vi "Match first tags ASCII and Unicode.vi"(6 "Type":T1, 9 "Hyperlink":string, 11 "Text":string) -> (1 "Array":T3(array[cluster]), 3 "Find tag ?":bool)   [LabVIEW 2019, in "Exaprom PDF.lvlib"]
doc: "Version 1.0\nDeveloped by Jean-Marc Simard\nCopyright © 2010, Exaprom Inc.\nAll rights reserved.\nLicense: BSD"
uses:
  Controls/Text Controls/Text type.ctl
  Controls/Text Controls/Unicode/Character type.ctl
  Exaprom PDF.lvlib
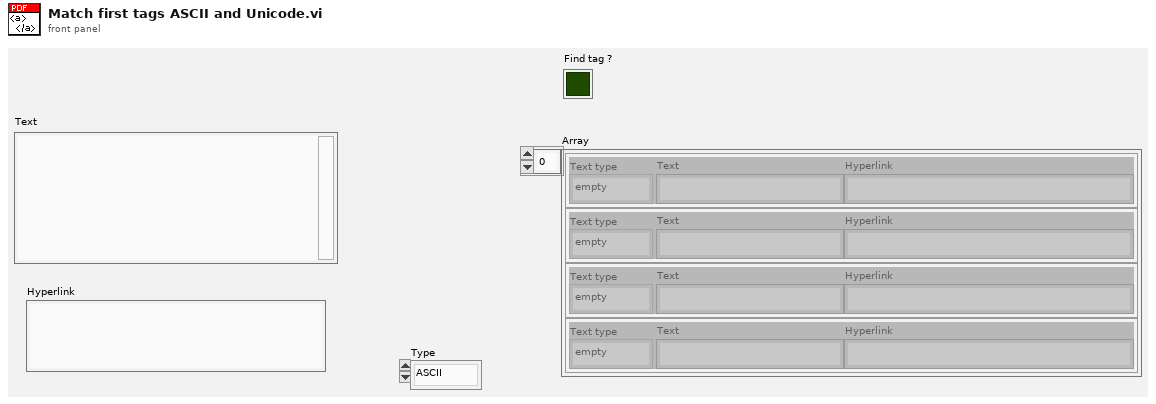
[diagram p1: front panel]
types:
  T1 = typedef "Exaprom PDF.lvlib/Character type.ctl" = enum16{"ASCII", "Unicode"}
  T2 = typedef "Exaprom PDF.lvlib/Text type.ctl" = enum16{"empty", "Text", "Hyperlink"}
  T3 = cluster{"Text type":T2, "Text":string, "Hyperlink":string}[]
  T4 = cluster{"Text type":T2, "Text type":T2, "Text type":T2}
  T5 = cluster{"Text type":T2, "Unicode String OUT":string, "Hyperlink":string}
  T6 = cluster{"Text type":T2, "Unicode String OUT":string, string}
  T7 = cluster{"Text type":T2, "Unicode String OUT":string, "Hyperlink":string}[]
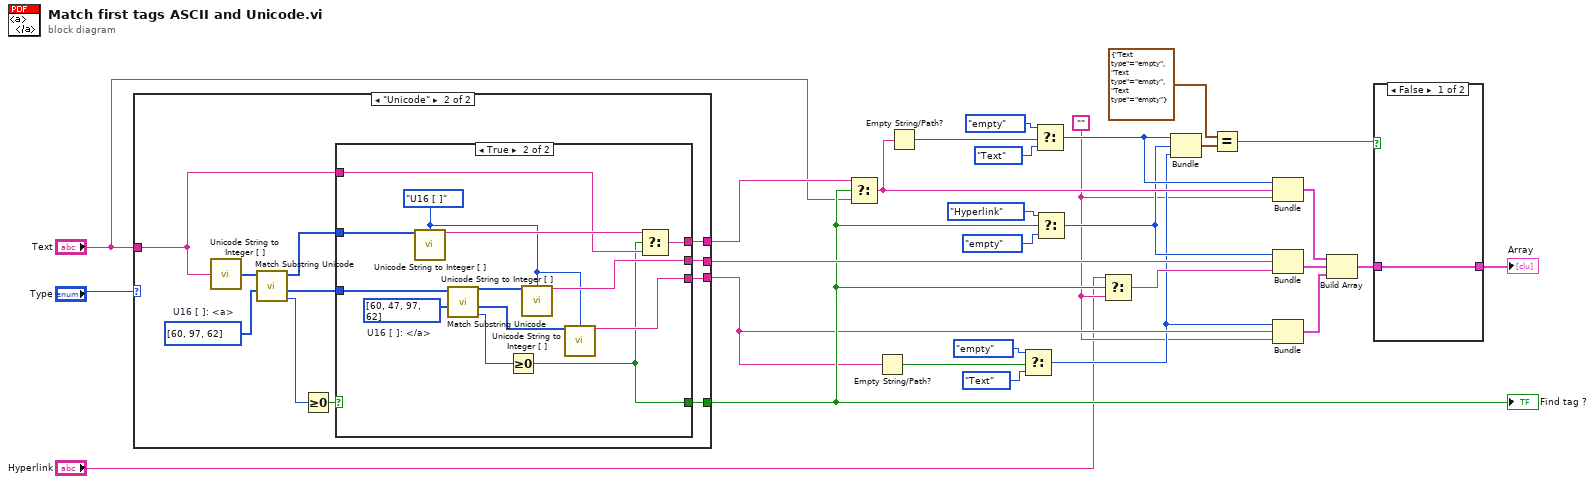
[diagram p0: block diagram]
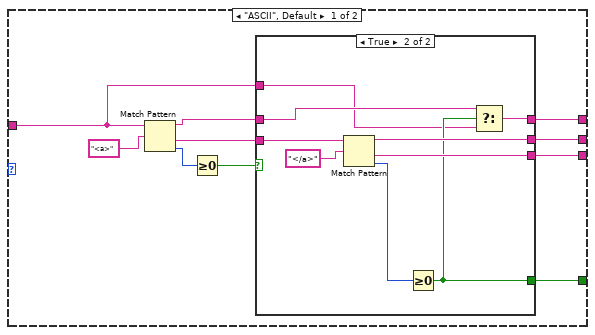
[diagram p2: hidden frame]
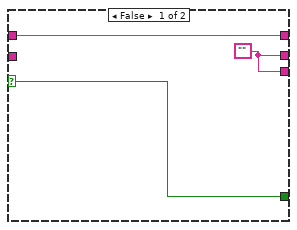
[diagram p3: hidden frame]
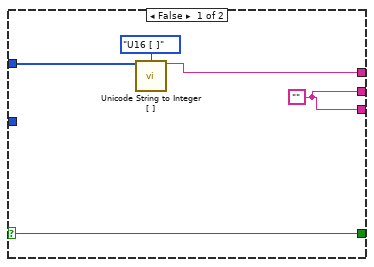
[diagram p4: hidden frame]
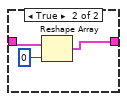
[diagram p5: hidden frame]
diagram:
  w4 = ""
  n1 = case shown="\"Unicode\"" "Type" {
    tunnel: [w34 w54] -> w29
    tunnel: [w33 w53] -> w24
    tunnel: [w32 w52] -> w18
    tunnel: [w31 w56] -> w13
    tunnel: "Text" -> [w30 w55]
    frame "ASCII", Default {
      n2 = Match Pattern(string=w30, regular expression="<a>") -> (before substring=w36:string, after substring=w35:string, offset past match=w39:i32)  [unwired: 2 out]
      n3 = Greater Or Equal To 0?(x=w39) -> (x >= 0?=w38:bool)
      n4 = case shown="True" w38 {
        selector: w38 -> [w40 _]
        tunnel: w36 -> [w42 w44]
        tunnel: [w42 w46] -> w33
        tunnel: w35 -> [_ w51]
        tunnel: [w41 w49] -> w34
        tunnel: [w41 w48] -> w31
        tunnel: [w40 w45] -> w32
        tunnel: w30 -> [_ w43]
        frame False {
          w41 = ""
        }
        frame True {
          n5 = Match Pattern(string=w51, regular expression="</a>") -> (before substring=w49:string, after substring=w48:string, offset past match=w47:i32)  [unwired: 2 out]
          n6 = Greater Or Equal To 0?(x=w47) -> (x >= 0?=w45:bool)
          n7 = Select(t=w44, s=w45, f=w43) -> (s? t:f=w46:string)
        }
      }
    }
    frame "Unicode" {
      w62 = u16[] [60, 97, 62]  # U16 [ ]: <a>
      n8 = call "Unicode String to Integer [ ].vi"("Unicode String"=w55) -> ("Char U16 [ ]"=w57:u16[])  [unwired: 12 in, 2 out]
      n9 = call "Match Substring Unicode.vi"("Substring (U16) [ ]"=w62, "String (U16) [ ]"=w57) -> ("offset past match"=w58:i32, "after substring"=w61:u16[], "before substring"=w60:u16[])  [unwired: 4 in, 1 out]
      n10 = Greater Or Equal To 0?(x=w58) -> (x >= 0?=w59:bool)
      n11 = case shown="True" w59 {
        selector: w59 -> [w66 _]
        tunnel: w60 -> [w64 w80]
        tunnel: w61 -> [_ w78]
        tunnel: w55 -> [_ w76]
        tunnel: [w63 w75] -> w53
        tunnel: [w67 w73] -> w54
        tunnel: [w67 w71] -> w56
        tunnel: [w66 w70] -> w52
        frame False {
          w67 = ""
          n12 = call "Unicode String to Integer [ ].vi"("Char U16 [ ] IN"=w64, "From"=enum16{"String", "U16 [ ]"}."U16 [ ]") -> ("Unicode String OUT"=w63:string)  [unwired: 11 in, 2 out]
        }
        frame True {
          w69 = u16[] [60, 47, 97, 62]  # U16 [ ]: </a>
          w68 = enum16{"String", "U16 [ ]"}."U16 [ ]" ("From")
          n13 = call "Unicode String to Integer [ ].vi"("Char U16 [ ] IN"=w80, "From"=w68) -> ("Unicode String OUT"=w79:string)  [unwired: 11 in, 2 out]
          n14 = call "Match Substring Unicode.vi"("Substring (U16) [ ]"=w69, "String (U16) [ ]"=w78) -> ("offset past match"=w77:i32, "after substring"=w72:u16[], "before substring"=w74:u16[])  [unwired: 4 in, 1 out]
          n15 = Greater Or Equal To 0?(x=w77) -> (x >= 0?=w70:bool)
          n16 = call "Unicode String to Integer [ ].vi"("Char U16 [ ] IN"=w74, "From"=w68) -> ("Unicode String OUT"=w73:string)  [unwired: 11 in, 2 out]
          n17 = call "Unicode String to Integer [ ].vi"("Char U16 [ ] IN"=w72, "From"=w68) -> ("Unicode String OUT"=w71:string)  [unwired: 11 in, 2 out]
          n18 = Select(t=w79, s=w70, f=w76) -> (s? t:f=w75:string)
        }
      }
    }
  }
  "Find tag ?" <- w18
  n19 = Select(t=w24, s=w18, f="Text") -> (s? t:f=w17:string)
  n20 = Empty String/Path?(string/path=w13) -> (empty?=w14:bool)
  n21 = Empty String/Path?(string/path=w17) -> (empty?=w23:bool)
  n22 = Select(t=Text_type."empty" ("Text type"), s=w14, f=Text_type."Text" ("Text type")) -> (s? t:f=w10:T2)
  n23 = Select(t=Text_type."empty" ("Text type"), s=w23, f=Text_type."Text" ("Text type")) -> (s? t:f=w12:T2)
  n24 = Select(t=Text_type."Hyperlink" ("Text type"), s=w18, f=Text_type."empty" ("Text type")) -> (s? t:f=w11:T2)
  n25 = Select(t="Hyperlink", s=w18, f=w4) -> (s? t:f=w28:string)
  n26 = Bundle("Text type"=w12, "Text type"=w11, "Text type"=w10) -> (w9:T4)  [unwired: 1 out]
  n27 = Equal?(x=T4 {"Text type"=enum."empty", "Text type"=enum."empty", "Text type"=enum."empty"}, y=w9) -> (x = y?=w7:bool)
  n28 = Bundle("Text type"=w12, "Text"=w17, w4) -> (w27:cluster{"Text type":T2, "Text":string, string})  [unwired: 1 out]
  n29 = Bundle("Text type"=w11, "Unicode String OUT"=w29, "Hyperlink"=w28) -> (w26:T5)  [unwired: 1 out]
  n30 = Bundle("Text type"=w10, "Unicode String OUT"=w13, w4) -> (w25:T6)  [unwired: 1 out]
  n31 = Build Array(w27, w26, w25) -> (w6:T7)
  n32 = case shown="False" w7 {
    tunnel: w6 -> [w81 w84]
    tunnel: [w81 w83] -> w5
    frame False {
    }
    frame True {
      n33 = Reshape Array(w84, 0 ("dimension size")) -> (w83:T7)
    }
  }
  "Array" <- w5
